vi "RefnumToLableValue_UTest.vi"() -> ()   [LabVIEW 2020]
panel:
  out "All the controls and their values":string="Double                        0                   \r\nInteger                       0                   \r\nBoolean                       False               \r\nString                                            \r\n"
  in  "String":string="Yeah!"
  in  "Boolean":bool
  in  "Integer":i32=3
  in  "Double":dbl=6.0
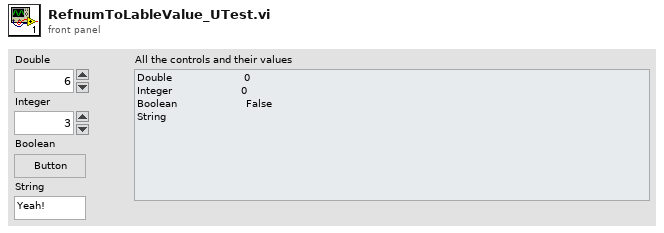
[diagram p1: front panel]
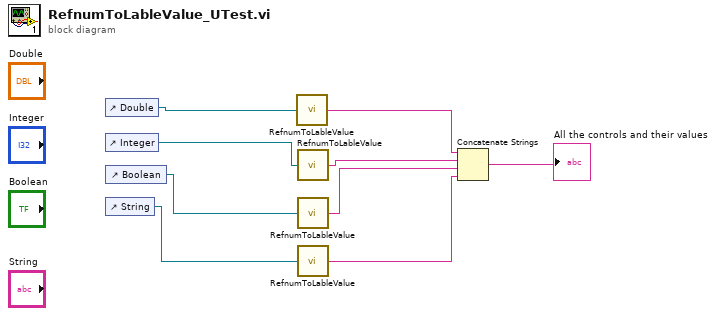
[diagram p0: block diagram]
diagram:
  n1 = control-ref of="Double"() -> (w9:refnum<vi>)
  n2 = control-ref of="Integer"() -> (w8:refnum<vi>)
  n3 = control-ref of="Boolean"() -> (w7:refnum<vi>)
  n4 = control-ref of="String"() -> (w6:refnum<vi>)
  n5 = call "RefnumToLableValue.vi"("Ctl Refnum"=w9) -> ("Control Lable Value String"=w5:string)
  n6 = call "RefnumToLableValue.vi"("Ctl Refnum"=w8) -> ("Control Lable Value String"=w4:string)
  n7 = call "RefnumToLableValue.vi"("Ctl Refnum"=w7) -> ("Control Lable Value String"=w3:string)
  n8 = call "RefnumToLableValue.vi"("Ctl Refnum"=w6) -> ("Control Lable Value String"=w2:string)
  n9 = Concatenate Strings(w5, w4, w3, w2) -> (→"All the controls and their values":string)
